vi "Settings Dialog.vi"(8 "error in (no error)":errorcluster, 11 "Settings in":T1={"Hardware Configuration"={"DAQmx AI Channels"="", "Max Input(V)"=0.0, "Min Input(V)"=0.0, "Input Sample Rate(Hz)"=0.0, "Input Samples"=0.0, "DAQmx Input Task"="", "DAQmx AO Channels"="", "Excitation Duty Cycle(%)"=0.0, "Excitation Current(Amps)"=0.0, "Max Output(Amps)"=0.0, "Min Output(Amps)"=0.0, "Output Sample Rate(Hz)"=0.0, "Output Samples"=0.0, "DAQmx Output Task"="", "Aquatrak COM Port"="", "DAQmx Ring Channel"="", "Ring Time Level Offset (V)"=0.0, "DAQmx Ring Time Task"="", "Thermistor Trigger Source"="", "Humidity Channel"="", "DAQmx Humidity Task"=""}, "Logging Configuration"={"Log File Base Path"=path "U:/Winston.Hensley/Documents/LabVIEW Data/Thermistor Data/Logged Data.log", "Data Log Refnum"=refnum}}) -> (0 "error out":errorcluster, 1 "Cancelled?":bool=TRUE, 2 "UI Refresh Needed?":bool, 3 "Settings out":T1={"Hardware Configuration"={"DAQmx AI Channels"="", "Max Input(V)"=0.0, "Min Input(V)"=0.0, "Input Sample Rate(Hz)"=0.0, "Input Samples"=0.0, "DAQmx Input Task"="", "DAQmx AO Channels"="", "Excitation Duty Cycle(%)"=0.0, "Excitation Current(Amps)"=0.0, "Max Output(Amps)"=0.0, "Min Output(Amps)"=0.0, "Output Sample Rate(Hz)"=0.0, "Output Samples"=0.0, "DAQmx Output Task"="", "Aquatrak COM Port"="", "DAQmx Ring Channel"="", "Ring Time Level Offset (V)"=0.0, "DAQmx Ring Time Task"="", "Thermistor Trigger Source"="", "Humidity Channel"="", "DAQmx Humidity Task"=""}, "Logging Configuration"={"Log File Base Path"=path "U:/Winston.Hensley/Documents/LabVIEW Data/Thermistor Data/Logged Data.log", "Data Log Refnum"=refnum}})   [LabVIEW 2018, in "Settings.lvlib"]
doc: "Dialog for selecting user specified settings."
uses:
  Settings.lvlib
  Settings.ctl
  Acquisition/Hardware Configuration.ctl
  Logging/Logging Configuration.ctl
  <vilib>/Utility/xml.llb/Write to XML File(string).vi
  Acquisition/Acquisition.lvlib
  Logging/Logging.lvlib
panel:
  in  "Thermistor Trigger Source":tag
  in  "Ring Time Cut-Off Level (V)":dbl
  in  "DAQmx Ring Channel":tag
  in  "Min Output(A)":dbl
  in  "Min Input(V)":dbl format="%#_3g"
  in  "Aquatrak COM Port":refnum<visa-resource-name>="COM1"
  in  "Max Output(A)":dbl
  in  "Excitation Current (A)":dbl
  in  "DAQmx Output Channels":tag
  in  "AI Sample Rate(Hz)":dbl
  in  "Input Samples":dbl
  in  "Max Input(V)":dbl
  in  "DAQmx Input Channels":tag
  in  "Log File Path":path
  in  "Cancel Button":bool
  in  "OK Button":bool
  # "Non visible portion of dialog (needed for connector pane)."
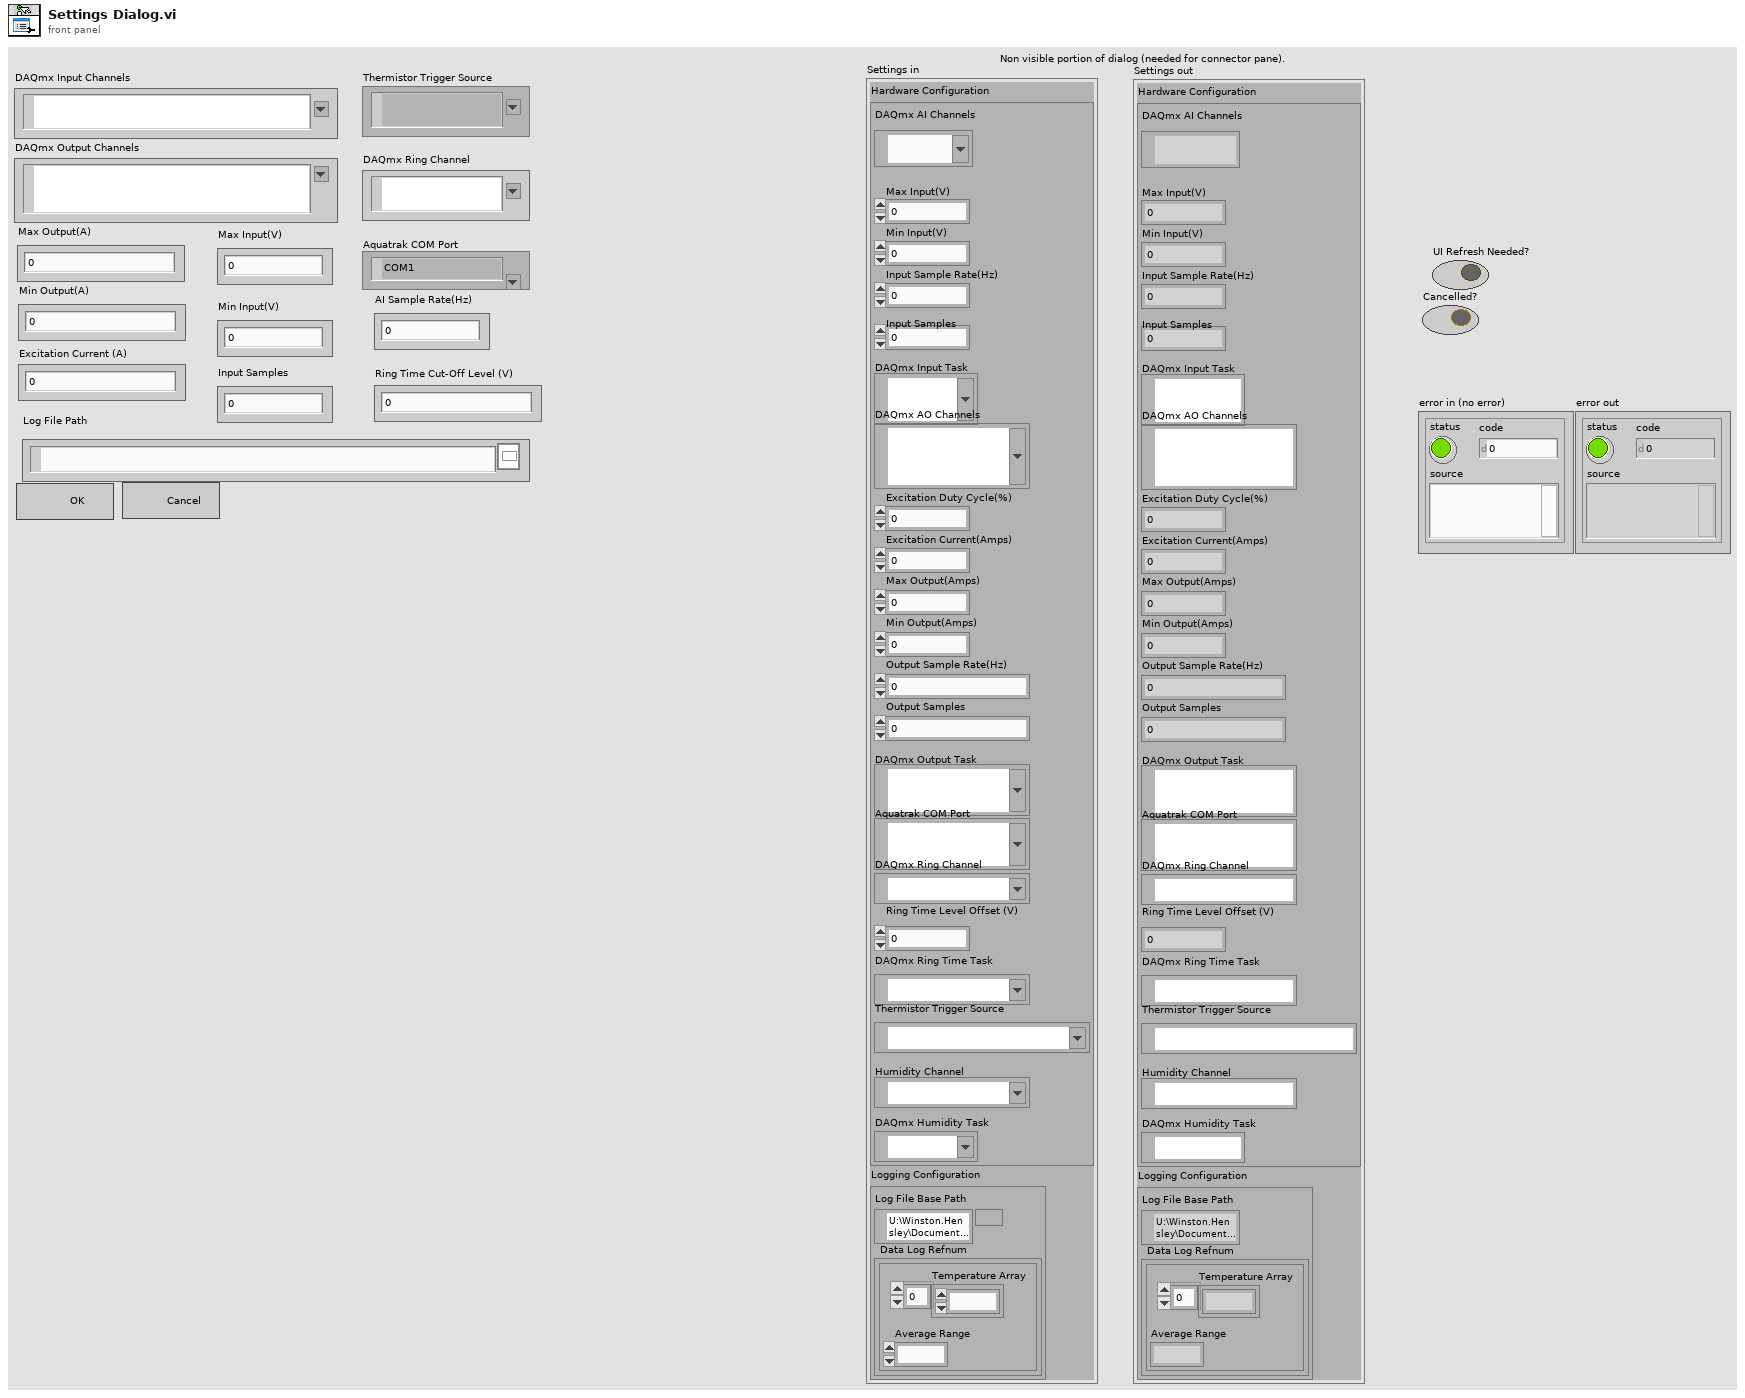
[diagram p1: front panel]
types:
  T1 = typedef "Settings.lvlib/Settings.ctl" = cluster{"Hardware Configuration":T2, "Logging Configuration":T3}
  T2 = typedef "Acquisition.lvlib/Hardware Configuration.ctl" = cluster{"DAQmx AI Channels":tag, "Max Input(V)":dbl, "Min Input(V)":dbl, "Input Sample Rate(Hz)":dbl, "Input Samples":dbl, "DAQmx Input Task":refnum<k21>, "DAQmx AO Channels":tag, "Excitation Duty Cycle(%)":dbl, "Excitation Current(Amps)":dbl, "Max Output(Amps)":dbl, "Min Output(Amps)":dbl, "Output Sample Rate(Hz)":dbl, "Output Samples":dbl, "DAQmx Output Task":refnum<k21>, "Aquatrak COM Port":refnum<visa-resource-name>, "DAQmx Ring Channel":tag, "Ring Time Level Offset (V)":dbl, "DAQmx Ring Time Task":refnum<k21>, "Thermistor Trigger Source":tag, "Humidity Channel":tag, "DAQmx Humidity Task":refnum<k21>}
  T3 = typedef "Logging.lvlib/Logging Configuration.ctl" = cluster{"Log File Base Path":path, "Data Log Refnum":refnum<k1>}
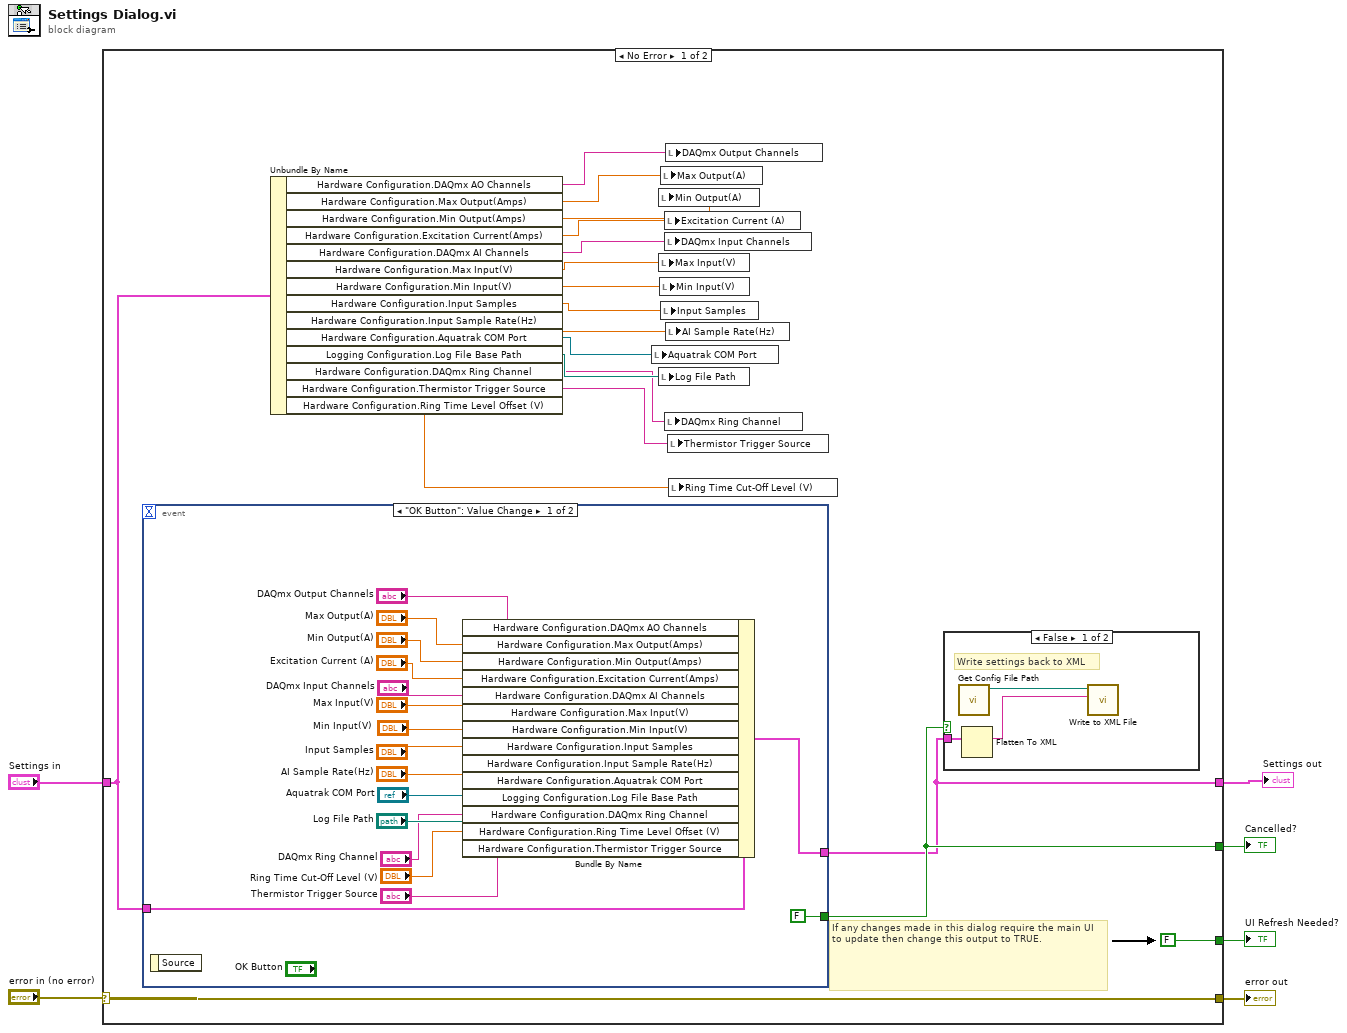
[diagram p0: block diagram]
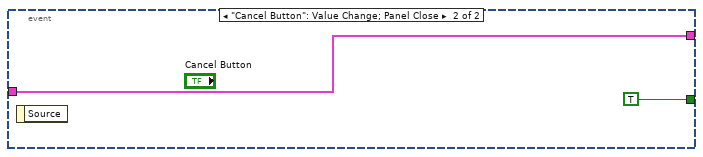
[diagram p3: hidden frame]
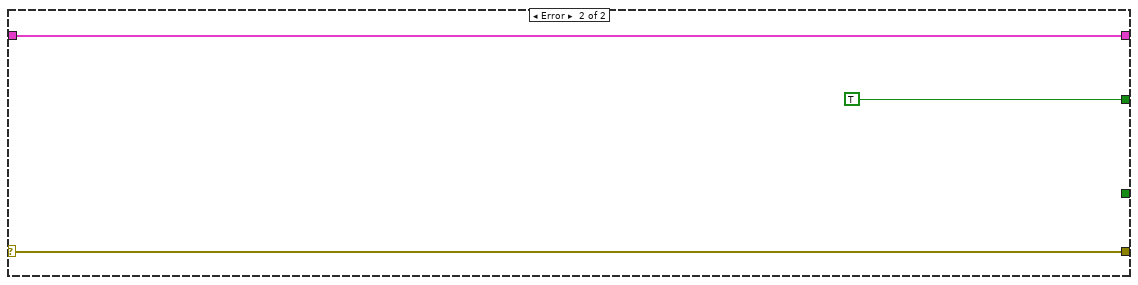
[diagram p4: hidden frame]
diagram:
  n1 = case shown="No Error" "error in (no error)" {
    selector: "error in (no error)" -> [w25 w50]
    tunnel: [w25 w50] -> w5
    tunnel: "Settings in" -> [w21 w49]
    tunnel: [w22 w49] -> w3
    tunnel: [FALSE ("UI Refresh Needed?") _] -> w2
    tunnel: [w23 TRUE ("UI Refresh Needed?")] -> w1
    frame No Error {
      # "If any changes made in this dialog require the main UI to update then change this output to TRUE."
      n2 = event shown="[0] \"OK Button\": Value Change" {
        selector: _ -> [_ _]
        dyn-events: _ -> [_ _]
        timeout: _ -> [_ _]
        tunnel: [w44 w47] -> w22
        tunnel: w21 -> [w36 w47]
        tunnel: [FALSE ("UI Refresh Needed?") TRUE ("UI Refresh Needed?")] -> w23
        event "OK Button": Value Change {
          n3 = event-data() -> ()  [unwired: 1 in, 1 out]
          n4 = Bundle By Name(cluster=w36, "Hardware Configuration.DAQmx AO Channels"="DAQmx Output Channels", "Hardware Configuration.Max Output(Amps)"="Max Output(A)", "Hardware Configuration.Min Output(Amps)"="Min Output(A)", "Hardware Configuration.Excitation Current(Amps)"="Excitation Current (A)", "Hardware Configuration.DAQmx AI Channels"="DAQmx Input Channels", "Hardware Configuration.Max Input(V)"="Max Input(V)", "Hardware Configuration.Min Input(V)"="Min Input(V)", "Hardware Configuration.Input Samples"="Input Samples", "Hardware Configuration.Input Sample Rate(Hz)"="AI Sample Rate(Hz)", "Hardware Configuration.Aquatrak COM Port"="Aquatrak COM Port", "Logging Configuration.Log File Base Path"="Log File Path", "Hardware Configuration.DAQmx Ring Channel"="DAQmx Ring Channel", "Hardware Configuration.Ring Time Level Offset (V)"="Ring Time Cut-Off Level (V)", "Hardware Configuration.Thermistor Trigger Source"="Thermistor Trigger Source") -> (w44:T1)
        }
        event "Cancel Button": Value Change; Panel Close {
          n5 = event-data() -> ()  [unwired: 1 in, 1 out]
        }
      }
      n6 = Unbundle By Name(w21) -> ("Hardware Configuration.DAQmx AO Channels"=w14:tag, "Hardware Configuration.Max Output(Amps)"=w11:dbl, "Hardware Configuration.Min Output(Amps)"=w10:dbl, "Hardware Configuration.Excitation Current(Amps)"=w15:dbl, "Hardware Configuration.DAQmx AI Channels"=w17:tag, "Hardware Configuration.Max Input(V)"=w18:dbl, "Hardware Configuration.Min Input(V)"=w12:dbl, "Hardware Configuration.Input Samples"=w19:dbl, "Hardware Configuration.Input Sample Rate(Hz)"=w20:dbl, "Hardware Configuration.Aquatrak COM Port"=w13:refnum<visa-resource-name>, "Logging Configuration.Log File Base Path"=w16:path, "Hardware Configuration.DAQmx Ring Channel"=w9:tag, "Hardware Configuration.Thermistor Trigger Source"=w7:tag, "Hardware Configuration.Ring Time Level Offset (V)"=w8:dbl)
      n7 = local write "Aquatrak COM Port"(w13) -> ()
      n8 = local write "Min Output(A)"(w10) -> ()
      n9 = local write "Max Input(V)"(w18) -> ()
      n10 = local write "Log File Path"(w16) -> ()
      n11 = local write "Min Input(V)"(w12) -> ()
      n12 = local write "Max Output(A)"(w11) -> ()
      n13 = local write "Input Samples"(w19) -> ()
      n14 = local write "Excitation Current (A)"(w15) -> ()
      n15 = local write "DAQmx Input Channels"(w17) -> ()
      n16 = local write "DAQmx Ring Channel"(w9) -> ()
      n17 = local write "DAQmx Output Channels"(w14) -> ()
      n18 = local write "AI Sample Rate(Hz)"(w20) -> ()
      n19 = local write "Thermistor Trigger Source"(w7) -> ()
      n20 = local write "Ring Time Cut-Off Level (V)"(w8) -> ()
      n21 = case shown="False" w23 {
        tunnel: w22 -> [w27 _]
        frame False {
          # "Write settings back to XML"
          n22 = call "Get Config File Path.vi"() -> ("XML File Path"=w28:path)  [unwired: 10 in, 1 out]
          n23 = Flatten To XML(anything=w27) -> (xml string=w26:string)
          n24 = call-poly <vilib>:"Write to XML File.vi"("XML Input"=w26, "XML File Path"=w28) -> ()  [unwired: 7 in, 3 out]
        }
        frame True {
        }
      }
    }
    frame Error {
    }
  }
  "UI Refresh Needed?" <- w2
  "error out" <- w5
  "Settings out" <- w3
  "Cancelled?" <- w1
